vi "printer com.vi"() -> ()   [LabVIEW 2018]
uses:
  <vilib>/Instr/_visa.llb/VISA Configure Serial Port (Instr).vi
panel:
  out "error out":errorcluster
  in  "VISA资源名称":refnum<visa-resource-name>
  out "读取缓冲区":string
  in  "停止":bool
  in  "发送":bool
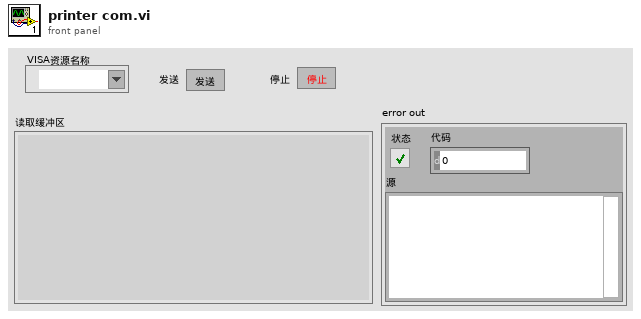
[diagram p1: front panel]
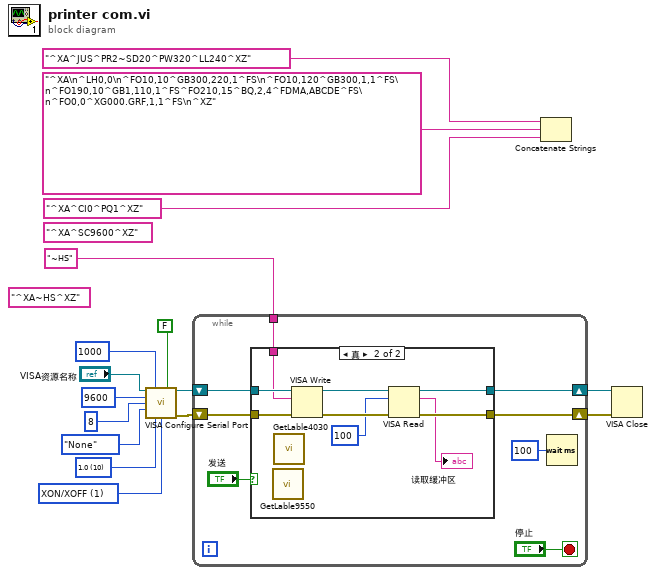
[diagram p0: block diagram]
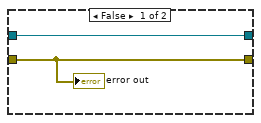
[diagram p2: hidden frame]
diagram:
  w1 = u16 1 items=["无", "XON/XOFF", "RTS/CTS", "XON/XOFF & RTS/CTS", "DTR/DSR", "XON/XOFF & DTR/DSR"] ("flow control (0:none)")
  (unwired) "^XA~HS^XZ"
  w3 = u16 10 items=["1.0"=10, "1.5"=15, "2.0"=20] ("stop bits (10: 1 bit)")
  (unwired) "^XA^SC9600^XZ"
  n1 = call-poly "VISA Configure Serial Port"("VISA resource name"="VISA资源名称", "timeout (10sec)"=u32 1000, "Enable Termination\nChar (T)"=FALSE ("Enable Termination\nChar (T)"), "baud rate (9600)"=u32 9600, "data bits (8)"=u16 8, "parity (0:none)"=enum16{"None", "Odd", "Even", "Mark", "Space"}."None", "stop bits (10: 1 bit)"=w3, "flow control (0:none)"=w1) -> ("VISA resource name out"=w16:refnum<visa-resource-name>, "error out"=w14:errorcluster)  [unwired: 6 in]
  n2 = while {
    shift-right: [w18] -> w15
    shift-left: w16 -> [w24]
    shift-right: [w17] -> w13
    shift-left: w14 -> [w23]
    tunnel: "~HS" -> [w19]
    stop <- "停止" stop-if-true
    n3 = case shown="真" "发送" {
      tunnel: w24 -> [w26 w35]
      tunnel: [w26 w31] -> w18
      tunnel: w23 -> [w25 w34]
      tunnel: [w25 w30] -> w17
      tunnel: w19 -> [_ w33]
      frame False {
        "error out" <- w25
      }
      frame True {
        n4 = call "GetLable9550.vi"() -> ()  [unwired: 1 in, 1 out]
        n5 = call "GetLable4030.vi"() -> ()  [unwired: 1 in, 1 out]
        n6 = VISA Write(VISA resource name=w35, write buffer=w33, error in (no error)=w34) -> (VISA resource name out=w32:refnum<visa-resource-name>, error out=w29:errorcluster)  [unwired: 1 out]
        n7 = VISA Read(VISA resource name=w32, byte count=u32 100 ("字节总数"), error in (no error)=w29) -> (VISA resource name out=w31:refnum<visa-resource-name>, read buffer=→"读取缓冲区":string, error out=w30:errorcluster)  [unwired: 1 out]
      }
    }
    n8 = Wait (ms)(milliseconds to wait=u32 100 ("等待时间（毫秒）")) -> ()  [unwired: 1 out]
  }
  n9 = Concatenate Strings("^XA^JUS^PR2~SD20^PW320^LL240^XZ", "^XA\n^LH0,0\n^FO10,10^GB300,220,1^FS\n^FO10,120^GB300,1,1^FS\n^FO190,10^GB1,110,1^FS^FO210,15^BQ,2,4^FDMA,ABCDE^FS\n^FO0,0^XG000.GRF,1,1^FS\n^XZ", "^XA^CI0^PQ1^XZ") -> ()  [unwired: 1 out]
  n10 = VISA Close(VISA resource name=w15, error in (no error)=w13) -> ()  [unwired: 1 out]
